vi "Exit.vi"(8 "error in (no error)":errorcluster, 11 "App ID in":u16) -> (0 "error out":errorcluster, 3 "App ID out":u16)   [LabVIEW 2018, in "TCPServer.lvlib"]
uses:
  TCPServer.lvlib
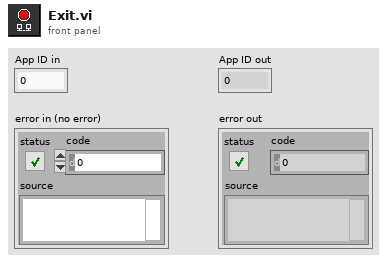
[diagram p1: front panel]
types:
  T1 = typedef "TCPServer.lvlib/App.ctl" = cluster{"Stack":refnum<queue>, "Cmd":cluster{"Conn":refnum<data-value>, "Daemon":refnum<vi>, "Counter":refnum<data-value>}, "Tlm":cluster{"Conn":refnum<data-value>, "Daemon":refnum<vi>, "Counter":refnum<data-value>}}
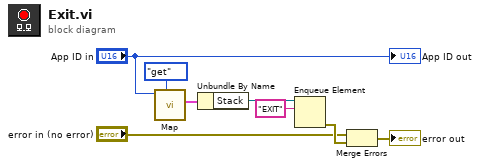
[diagram p0: block diagram]
diagram:
  n1 = call "Map.vi"("Action"=enum8{"noop", "get", "set", "pop"}."get", "App ID in"="App ID in") -> ("App out"=w1:T1)  [unwired: 7 in, 2 out]
  n2 = Unbundle By Name(w1) -> ("Stack"=w8:refnum<queue>)
  n3 = Enqueue Element(queue=w8, element="EXIT") -> (error out=w6:errorcluster)  [unwired: 2 in, 2 out]
  n4 = Merge Errors("error in (no error)", w6) -> (→"error out":errorcluster)
  "App ID out" <- "App ID in"
